vi "Set Segment Remap.vi"(8 "Error In":errorcluster, 10 "Segment Remap":enum8{"COL 0 -> SEG0", "COL127 -> SEG0"}(ring), 11 "LINX Resource":T1) -> (0 "Error Out":errorcluster, 3 "LINX Resource":T1)   [LabVIEW 2014, in "LMH-LINX.lvlib" / "SSD1306.lvlib"]
doc: "Configure the SSD1306's segment remapping."
uses:
  SSD1306.lvlib
  Private/Type Defs/LINX Ref.ctl
  Private/Type Defs/Platform.ctl
  Private/Type Defs/Interface.ctl
  Private/Device/Type Defs/LINX Device Config.ctl
  Private/Device/Type Defs/TCP Config.ctl
  Private/Device/Type Defs/Channels.ctl
  Private/SSD1306 FGV State.ctl
  Peripherals/SPI/SPI CS Config.ctl
  Private/Type Defs/Peripherals/SPI/SPI CS Logic Level.ctl
  Peripherals/Digital/Digital Write 1 Chan.vi
  Peripherals/SPI/SPI Write Read 1 Frame.vi
  LMH-LINX.lvlib
  Private/Device/Device.lvlib
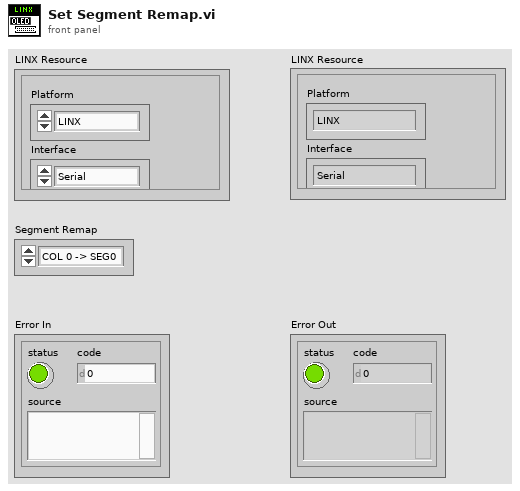
[diagram p1: front panel]
types:
  T1 = typedef "LMH-LINX.lvlib/LINX Ref.ctl" = cluster{"Platform":T2, "Interface":T3, "LINX Device Config":T4}
  T2 = typedef "LMH-LINX.lvlib/Platform.ctl" = enum16{"LINX", "myRIO"}
  T3 = typedef "LMH-LINX.lvlib/Interface.ctl" = enum16{"Serial", "TCP"}
  T4 = typedef "LMH-LINX.lvlib/Device.lvlib/LINX Device Config.ctl" = cluster{"Interface":T3, "COM Port":refnum<visa-resource-name>, "TCP Configuration":T5, "Device Family":u8, "Device ID":u8, "Device Name":string, "TCP Ref":refnum<k5>, "Channels":T6}
  T5 = typedef "LMH-LINX.lvlib/Device.lvlib/TCP Config.ctl" = cluster{"IP Address":string, "Port":u16}
  T6 = typedef "LMH-LINX.lvlib/Channels.ctl" = cluster{"DI":u8[], "DO":u8[], "AI":u8[], "AO":u8[], "PWM":u8[], "QE":u8[], "UART":u8[], "I2C 2":u8[], "SPI":u8[], "CAN":u8[], "Servo":u8[], "AI Ref (V)":dbl, "AO Ref (V)":dbl, "AO Resolution (Bits)":u8}
  T7 = typedef "LMH-LINX.lvlib/SPI CS Config.ctl" = cluster{"CS Channel":u8, "CS Logic Level":T8}
  T8 = typedef "LMH-LINX.lvlib/SPI CS Logic Level.ctl" = enum8{"Active Low", "Active High"}
  T9 = typedef "LMH-LINX.lvlib/SSD1306.lvlib/SSD1306 FGV State.ctl" = enum16{"Init", "Set", "Get"}
  T10 = typedef "LMH-LINX.lvlib/SSD1306.lvlib/SSD1306 Config.ctl" = cluster{"SPI Channel (0)":u8, "VDD Channel":u8, "VBAT Channel":u8, "RESET Channel":u8, "DC Channel":u8, "SPI CS (3)":u8}
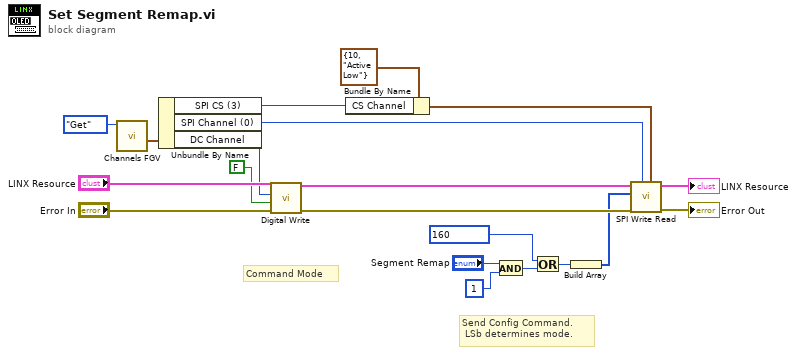
[diagram p0: block diagram]
diagram:
  # "Send Config Command. \n LSb determines mode."
  # "Command Mode"
  n1 = call "Channels FGV.vi"("SSD1306 FGV State"=SSD1306_FGV_State."Get") -> ("SSD1306 Channels"=w17:T10)  [unwired: 10 in]
  n2 = Unbundle By Name(w17) -> ("SPI CS (3)"=w2:u8, "SPI Channel (0)"=w4:u8, "DC Channel"=w16:u8)
  n3 = call-poly "Digital Write.vi"("Error In"="Error In", "Output Value"=FALSE, "DO Channel"=w16, "LINX Resource"="LINX Resource") -> ("Error Out"=w6:errorcluster, "LINX Resource"=w7:T1)  [unwired: 6 in]
  n4 = Bundle By Name(cluster=T7 {"CS Channel"=10, "CS Logic Level"=enum."Active Low"} ("CS Configuration"), "CS Channel"=w2) -> (w1:T7)
  n5 = And(x="Segment Remap", y=u8 1) -> (x .and. y?=w12:u8)
  n6 = Or(x=u8 160, y=w12) -> (x .or. y?=w10:u8)
  n7 = Build Array(w10) -> (w5:u8[])
  n8 = call-poly "SPI Write Read.vi"("CS Configuration"=w1, "SPI Channel (0)"=w4, "Error In"=w6, "Data"=w5, "LINX Resource"=w7) -> ("Error Out"=→"Error Out":errorcluster, "LINX Resource"=→"LINX Resource":T1)  [unwired: 4 in, 1 out]
